vi "3D Model Controll (SubVI).vi"(8 "error in (no error)":errorcluster, 9 "Numeric":i32, 10 "Numeric 2":i32, 11 "SceneObject in":refnum<vi>) -> (3 "SceneNode out":refnum<vi>(3d-picture))   [LabVIEW 2012]
uses:
  <vilib>/Utility/miscctls.llb/LV3DPointTypeDef.ctl
  <vilib>/picture/3D Picture Control/NI_3D Picture Control.lvlib
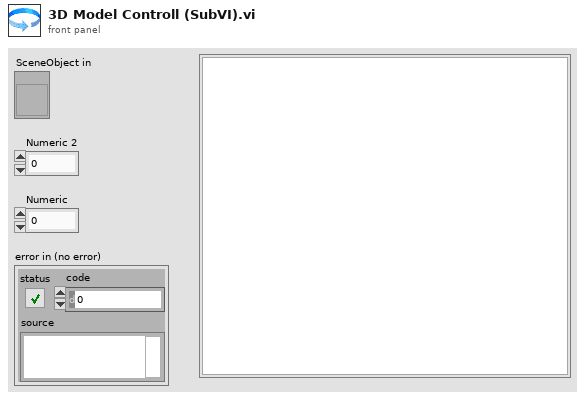
[diagram p1: front panel]
types:
  T1 = typedef "LV3DPointTypeDef.ctl" = cluster{"X":sgl, "Y":sgl, "Z":sgl}
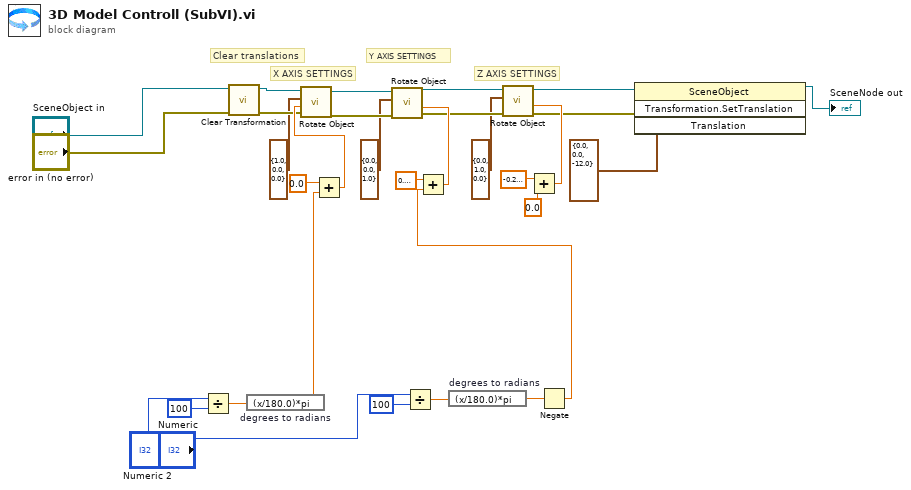
[diagram p0: block diagram]
diagram:
  # "Z AXIS SETTINGS"
  # "Y AXIS SETTINGS"
  # "Clear translations"
  # "X AXIS SETTINGS"
  n1 = Divide(x="Numeric 2", y=100) -> (x/y=w22:dbl)
  n2 = call <vilib>:"Clear Transformation.vi"("error in (no error)"="error in (no error)", "Object Refnum In"="SceneObject in") -> ("error out"=w12:errorcluster, "Object Refnum Out"=w2:refnum<vi>)  [unwired: 8 out]
  n3 = expression code="(x/180.0)*pi" "degrees to radians"(w22) -> (w26:dbl)
  n4 = Add(x=sgl 0.0 ("default X"), y=w26) -> (x+y=w14:dbl)
  n5 = call <vilib>:"Rotate Object.vi"("error in (no error)"=w12, "Angle"=w14, "Axis"=cluster{"X":sgl, "Y":sgl, "Z":sgl} {"X"=1.0, "Y"=0.0, "Z"=0.0}, "Scene.Object In"=w2) -> ("error out"=w11:errorcluster, "Scene.Object Out"=w10:refnum<vi>)  [unwired: 6 out]
  n6 = Divide(x="Numeric", y=100) -> (x/y=w28:dbl)
  n7 = expression code="(x/180.0)*pi" "degrees to radians"(w28) -> (w30:dbl)
  n8 = Add(x=sgl -0.2 ("Z"), y=sgl 0.0) -> (x+y=w19:sgl)
  n9 = Negate(x=w30) -> (-x=w31:dbl)
  n10 = Add(x=sgl 0.6 ("default Y"), y=w31) -> (x+y=w17:dbl)
  n11 = call <vilib>:"Rotate Object.vi"("error in (no error)"=w11, "Angle"=w17, "Axis"=cluster{"X":sgl, "Y":sgl, "Z":sgl} {"X"=0.0, "Y"=0.0, "Z"=1.0}, "Scene.Object In"=w10) -> ("error out"=w9:errorcluster, "Scene.Object Out"=w8:refnum<vi>)  [unwired: 6 out]
  n12 = call <vilib>:"Rotate Object.vi"("error in (no error)"=w9, "Angle"=w19, "Axis"=cluster{"X":sgl, "Y":sgl, "Z":sgl} {"X"=0.0, "Y"=1.0, "Z"=0.0}, "Scene.Object In"=w8) -> ("error out"=w7:errorcluster, "Scene.Object Out"=w6:refnum<vi>)  [unwired: 6 out]
  n13 = invoke class="SceneObject" method="Transformation.SetTranslation"(reference=w6, error in=w7, "Translation"=T1 {"X"=0.0, "Y"=0.0, "Z"=-12.0}) -> (reference out=→"SceneNode out":refnum<vi>)  [unwired: 1 in, 3 out]
